vi "MathCad_App_Open_New_Reference.vi"(8 "error in (no error)":errorcluster, 10 "Visible":bool=TRUE, 11 "open new instance":bool) -> (0 "error out (no error)":errorcluster, 3 "IMathcadApp Ref":refnum<k7>)   [LabVIEW 2015]
doc: "Opens a Mathcad Application. \n\nInputs\n\nVisible - If true then the Mathcad Application User Interface is visible.\nOpen New Instance- If true opens a new instance of the Application, otherwise returns a reference to the one open. If false and no Mathcad Applications are running, opens a new reference.\n\nOutputs\n\nIMathcadApp Ref- Reference to the Mathcad Application Class"
panel:
  in  "Mathcad.IMathcadApplicatio  Reference In":refnum<k7>
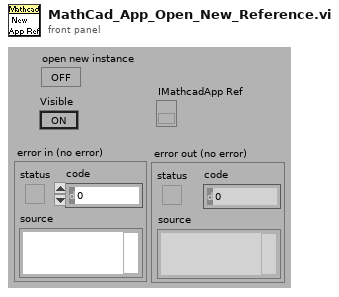
[diagram p1: front panel]
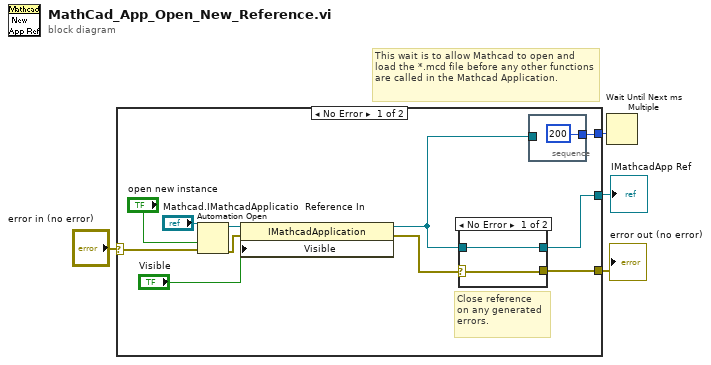
[diagram p0: block diagram]
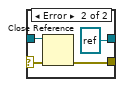
[diagram p2: hidden frame]
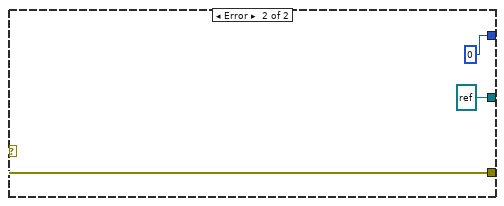
[diagram p3: hidden frame]
diagram:
  # "This wait is to allow Mathcad to open and load the *.mcd file before any other functions are called in the Mathcad Application."
  n1 = case shown="No Error" "error in (no error)" {
    selector: "error in (no error)" -> [w9 w24]
    tunnel: [w6 w24] -> w4
    tunnel: [w10 u32 0 ("millisecond multiple")] -> w3
    tunnel: [w7 refnum<k7> refnum] -> w2
    frame No Error {
      # "Close reference\non any generated\nerrors."
      n2 = Automation Open(error in (no error)=w9, Automation Refnum="Mathcad.IMathcadApplicatio  Reference In", 9:"open new instance") -> (Automation Refnum=w13:refnum<k7>, error out=w12:errorcluster)  [unwired: 1 in]
      n3 = property class="IMathcadApplication"(reference=w13, error in=w12, "Visible"="Visible") -> (reference out=w5:refnum<k7>, error out=w8:errorcluster)
      n4 = case shown="No Error" w8 {
        selector: w8 -> [w17 w19]
        tunnel: w5 -> [w18 w22]
        tunnel: [w18 refnum<k7> refnum ("IMathcadApp Ref")] -> w7
        tunnel: [w17 w20] -> w6
        frame No Error {
        }
        frame Error {
          n5 = Close Reference(reference=w22, error in (no error)=w19) -> (error out=w20:errorcluster)
        }
      }
      n6 = stacked-sequence {
        tunnel: [u32 200 ("millisecond multiple")] -> w10
        tunnel: w5 -> [_]
        frame #0 {
        }
      }
    }
    frame Error {
    }
  }
  "error out (no error)" <- w4
  "IMathcadApp Ref" <- w2
  n7 = Wait Until Next ms Multiple(millisecond multiple=w3) -> ()  [unwired: 1 out]
